vi "Analog DAQ_Connect.vi"(0 "Instance Inbox Address":string, 11 "error in (no error)":errorcluster) -> (4 "Analog DAQ Out":refnum<class "FTW-ActorConnector.lvclass">, 15 "error out":errorcluster)   [LabVIEW 2018]
uses:
  source/actor/Connector/FTW-ActorConnector.lvclass
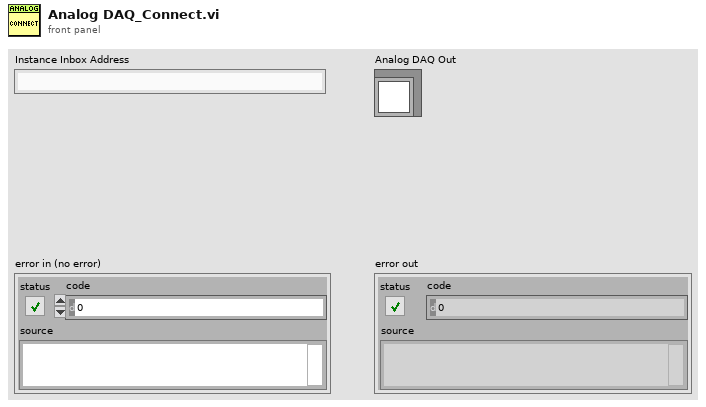
[diagram p1: front panel]
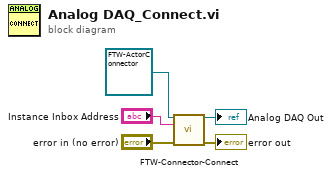
[diagram p0: block diagram]
diagram:
  n1 = call-dynamic "FTW-Connector-Connect.vi"("FTW Actor Connector Type"=refnum<class "FTW-ActorConnector.lvclass"> refnum ("Actor Template In"), "Instance Inbox Address"="Instance Inbox Address", "error in"="error in (no error)") -> ("FTW Actor Connector"=→"Analog DAQ Out":refnum<class "FTW-ActorConnector.lvclass">, "error out"=→"error out":errorcluster)  [unwired: 11 in]
